vi "Read DigitalVariable Setups from Ini.vi"(0 "error in (no error)":errorcluster, 1 "Path":path, 7 "Enum with Variable List":variant, 12 "Section(\"Default\")":string="Default") -> (4 "error out":errorcluster, 8 "Digitale User settigns":T1[](array[typedef]))   [LabVIEW 2011]
uses:
  User Setting DigitalChannel.ctl
  Alarm Responce.ctl
  Action List.ctl
  Alarm Responce dig.ctl
  <vilib>/Utility/VariantDataType/GetNumericInfo.vi
  <vilib>/Utility/libraryn.llb/Check if File or Folder Exists.vi
  <vilib>/Utility/config.llb/NI_LVConfig.lvlib
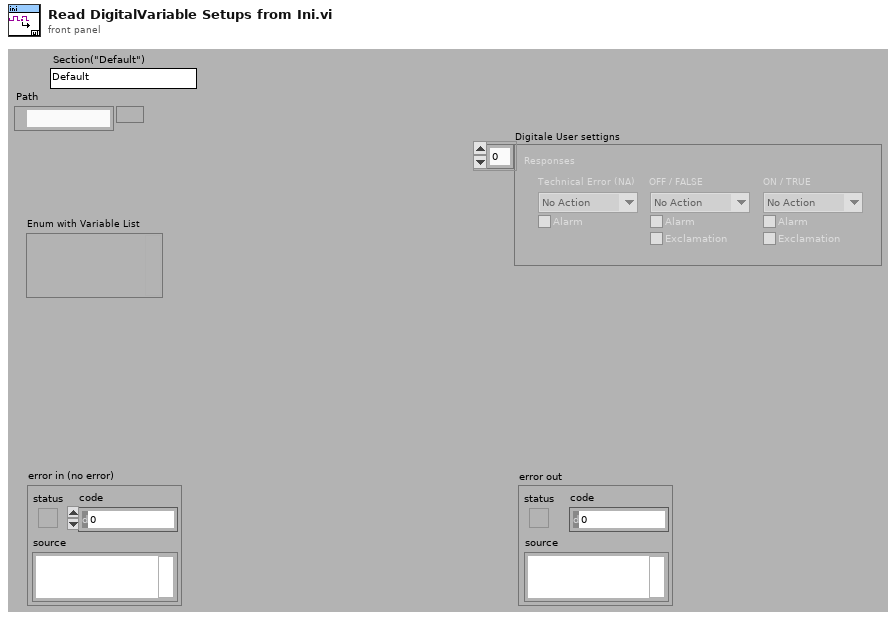
[diagram p1: front panel]
types:
  T1 = typedef "User Setting DigitalChannel.ctl" = cluster{"Responses":cluster{"Technical Error (NA)":T2, "OFF / FALSE":T4, "ON / TRUE":T4}}
  T2 = typedef "Alarm Responce.ctl" = cluster{"Action":T3, "Alarm":bool}
  T3 = typedef "Action List.ctl" = enum16{"No Action", "Stop Motor", "Turn Off HV"}
  T4 = typedef "Alarm Responce dig.ctl" = cluster{"Action":T3, "Alarm":bool, "Exclamation":bool}
  T5 = typedef "NI_LVConfig.lvlib/Config Data RefNum.ctl" = refnum<k1>
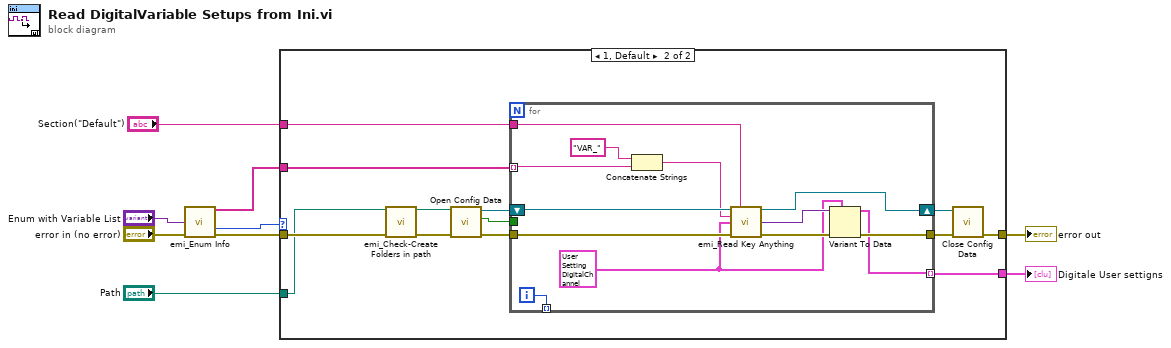
[diagram p0: block diagram]
diagram:
  n1 = call "emi_Enum Info.vi"("Enum"="Enum with Variable List", "error in (no error)"="error in (no error)") -> ("Text Elements"=w6:string[], "Numb Elements"=w7:i32, "error out"=w4:errorcluster)  [unwired: 10 in, 1 out]
  n2 = case shown="1, Default" w7 {
    tunnel: w6 -> [_ w21]
    tunnel: w4 -> [w10 w13]
    tunnel: [w10 w18] -> w9
    tunnel: [_ w17] -> w1
    tunnel: "Path" -> [_ w12]
    tunnel: "Section(\"Default\")" -> [_ w14]
    frame 0 {
    }
    frame 1, Default {
      n3 = call "emi_Check-Create Folders in path.vi"("Path including file"=w12, "error in (no error)"=w13) -> ("Path out"=w15:path, "error out"=w16:errorcluster)  [unwired: 11 in, 1 out]
      n4 = call <vilib>:"Open Config Data.vi"("error in (no error)"=w16, "configuration file path"=w15) -> ("error out"=w23:errorcluster, "file created?"=w11:bool, "refnum"=w22:T5)  [unwired: 7 in]
      n5 = for {
        tunnel: w21 -> [w27] mode=indexing
        tunnel: w23 -> [w35]
        tunnel: w14 -> [w34]
        tunnel: [w30] -> w20
        shift-right: [w29] -> w19
        shift-left: w22 -> [w33]
        tunnel: [w28] -> w17 mode=indexing
        tunnel: [w26] -> _ mode=indexing
        tunnel: w11 -> [_]
        i -> [w26]
        w24 = T1 {"Responses"={"Technical Error (NA)"={"Action"=enum."No Action", "Alarm"=FALSE}, "OFF / FALSE"={"Action"=enum."No Action", "Alarm"=FALSE, "Exclamation"=FALSE}, "ON / TRUE"={"Action"=enum."No Action", "Alarm"=FALSE, "Exclamation"=FALSE}}} ("User settings")
        n6 = Concatenate Strings("VAR_" ("string"), w27) -> (w31:string)
        n7 = call "emi_Read Key Anything.vi"("Ini file refnum"=w33, "Section(Default)"=w34, "Name"=w31, "Anything"=w24, "error in (no error)"=w35) -> ("Ini file refnum out"=w29:T5, "Anything Out"=w25:variant, "error out"=w32:errorcluster)  [unwired: 7 in, 1 out]
        n8 = Variant To Data(error in=w32, type=w24, Variant=w25) -> (data=w28:T1, error out=w30:errorcluster)
      }
      n9 = call <vilib>:"Close Config Data.vi"("error in (no error)"=w20, "refnum"=w19) -> ("error out"=w18:errorcluster)  [unwired: 8 in, 1 out]
    }
  }
  "Digitale User settigns" <- w1
  "error out" <- w9
